vi "U3 Stream Simple Example.vi"() -> ()   [LabVIEW 2021]
panel:
  in  "Scan List (-)":u8[](array[numeric])=[31, 31, 31, 31, 31, 31, 31, 31, 31, 31, 31, 31, 31, 31, 31, 31, 31, 31, 31, 31, 31, 31, 31, 31, 31, 31, 31, 31, 31, 31, 31, 31, 31, 31, 31, 31, 31, 31, 31, 31, 31, 31, 31, 31, 31, 31, 31, 31, 31, 31, 31, 31, 31, 31, 31, 31, 31, 31, 31, 31, 31, 31, 31, 31, 31, 31, 31, 31, 31, 31, 31, 31, 31, 31, 31, 31, 31, 31, 31, 31, 31, 31, 31, 31, 31, 31, 31, 31, 31, 31, 31, 31, 31, 31, 31, 31, 31, 31, 31, 31, 31, 31, 31, 31, 31, 31, 31, 31, 31, 31, 31, 31, 31, 31, 31, 31, 31, 31, 31, 31, 31, 31, 31, 31, 31, 31, 31, 31]
  out "Waveform Graph":dbl[][](graph)
  in  "Scan List (+)":u8[](array[numeric])=[0, 1, 2, 3]
  out "Actual Scan Rate (Hz)":dbl=1000.0 format="%.3f"
  out "# Scans Read":i32
  out "# of iterations":i32
  out "Data":dbl[][](array[numeric]) format="%.3f"
  in  "Scan Rate (Hz)":dbl=1000.0 format="%.3f"
  in  "stop":bool
  out "Error Message":string
  # "This example streams from the first found USB U3.  Streaming\nrequires U3 hardware revision 1.21+."
  # "The + scan list is the positive\nchannels.  For each element in\nthe + list, there must also be\nan element in the - list, which is\nthe negative channels.  For\nsingle-ended channels, put in\n31 for the negative channel."
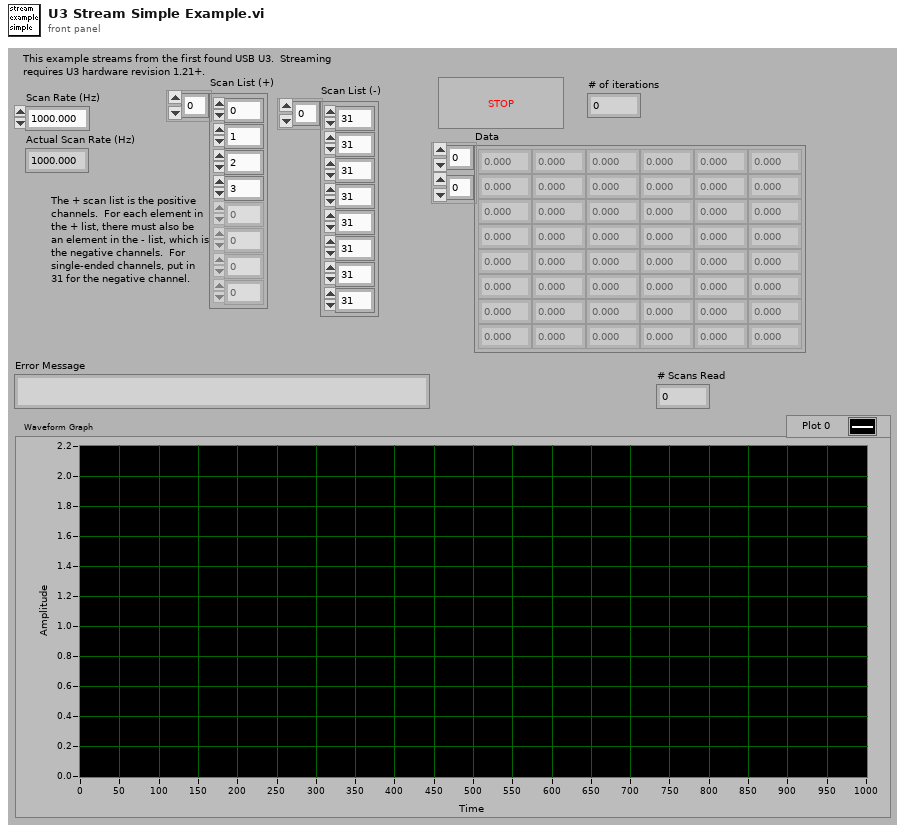
[diagram p1: front panel]
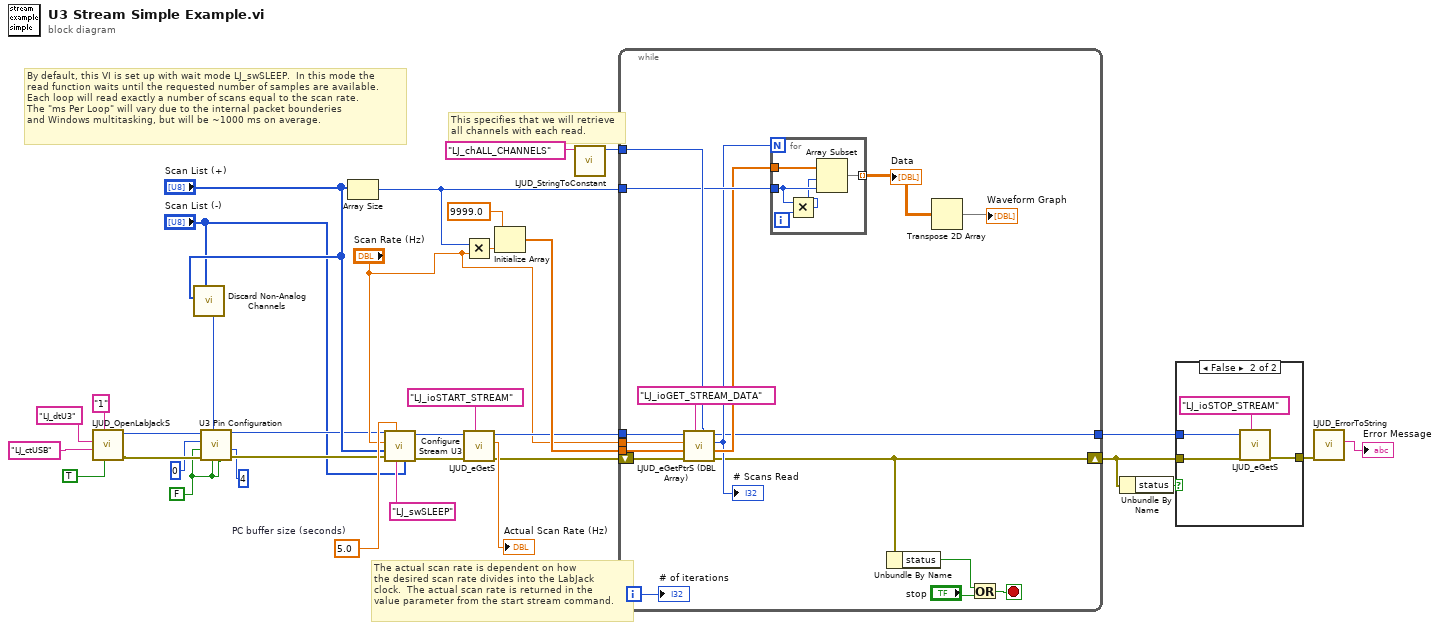
[diagram p0: block diagram]
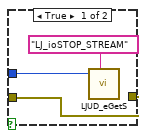
[diagram p2: hidden frame]
diagram:
  w11 = FALSE ("Enable DAC1")
  w24 = 5.0  # PC buffer size (seconds)
  # "This specifies that we will retrieve\nall channels with each read."
  # "The actual scan rate is dependent on how\nthe desired scan rate divides into the LabJack\nclock.  The actual scan rate is returned in the\nvalue parameter from the start stream command."
  # "By default, this VI is set up with wait mode LJ_swSLEEP.  In this mode the\nread function waits until the requested number of samples are available.\nEach loop will read exactly a number of scans equal to the scan rate.\nThe \"ms Per Loop\" will vary due to the internal packet bounderies\nand Windows multitasking, but will be ~1000 ms on average."
  n1 = call "LJUD_OpenLabJackS.vi"("FirstFound"=TRUE, "Address"="1", "ConnectionType"="LJ_ctUSB", "DeviceType"="LJ_dtU3") -> ("error out"=w14:errorcluster, "Handle"=w15:i32)  [unwired: 5 in, 1 out]
  n2 = call "Discard Non-Analog Channels.vi"("Channels In (-)"="Scan List (-)", "Channels In"="Scan List (+)") -> ("FIO/EIO Analog Enable"=w10:i32)  [unwired: 6 in, 3 out]
  n3 = call "U3 Pin Configuration.vi"("Timer/Counter Pin Offset"=u8 4, "Enable Counter1"=w11, "Enable Counter0"=w11, "FIO/EIO Analog Enable"=w10, "error in"=w14, "Enable DAC1"=w11, "Number of Timers Enabled"=u8 0, "Handle In"=w15) -> ("error out"=w7:errorcluster, "Handle Out"=w8:i32)  [unwired: 2 in]
  n4 = Array Size(array="Scan List (+)") -> (size(s)=w28:i32)
  n5 = call "Configure Stream U3.vi"("Scan List (-)"="Scan List (-)", "Wait Mode"="LJ_swSLEEP" ("Wait Mode (2)"), "PC buffer size (seconds)"=w24, "error in"=w7, "Scan List (+)"="Scan List (+)", "Scan Rate (Hz)"="Scan Rate (Hz)", "Handle In"=w8) -> ("error out"=w32:errorcluster, "Handle Out"=w33:i32)  [unwired: 2 in, 1 out]
  n6 = Multiply(x=w28, y="Scan Rate (Hz)") -> (x*y=w31:dbl)
  n7 = call "LJUD_eGetS.vi"("IOType"="LJ_ioSTART_STREAM", "error in"=w32, "Handle In"=w33) -> ("error out"=w17:errorcluster, "Value Read"=→"Actual Scan Rate (Hz)":dbl, "Handle Out"=w22:i32)  [unwired: 6 in]
  n8 = Initialize Array(9999.0, w31) -> (w29:dbl[])
  n9 = call "LJUD_StringToConstant.vi"("String"="LJ_chALL_CHANNELS") -> ("Constant Number"=w18:i32)  [unwired: 9 in, 1 out]
  n10 = while {
    tunnel: [w35] -> w4
    shift-left: w17 -> [w42]
    shift-right: [w36] -> w16
    tunnel: w18 -> [w43]
    tunnel: w28 -> [w39]
    tunnel: w29 -> [w46]
    tunnel: "Scan Rate (Hz)" -> [w45]
    tunnel: w22 -> [w48]
    i -> [w44]
    stop <- w49 stop-if-true
    n11 = call "LJUD_eGetPtrS (DBL Array).vi"("Channel"=w43, "IOType"="LJ_ioGET_STREAM_DATA", "error in"=w42, "DBL Array Write"=w46, "Value"=w45, "Handle In"=w48) -> ("error out"=w36:errorcluster, "DBL Array Read"=w38:dbl[], "Value"=w37:i32, "Handle Out"=w35:i32)  [unwired: 2 in]
    "# Scans Read" <- w37
    n12 = for {
      N: w37 -> [_]
      tunnel: w38 -> [w56]
      tunnel: w39 -> [w55]
      tunnel: [w52] -> w40 mode=indexing
      i -> [w54]
      n13 = Multiply(x=w55, y=w54) -> (x*y=w53:i32)
      n14 = Array Subset(array=w56, index=w53, length=w55) -> (w52:dbl[])
    }
    "Data" <- w40
    n15 = Unbundle By Name(w36) -> ("status"=w50:bool)
    n16 = Transpose 2D Array(2D array=w40) -> (transposed array=→"Waveform Graph":dbl[][])
    n17 = Or(x=w50, y="stop") -> (x .or. y?=w49:bool)
    "# of iterations" <- w44
  }
  n18 = Unbundle By Name(w16) -> ("status"=w20:bool)
  n19 = case shown="False" w20 {
    tunnel: [w58 w62] -> w26
    tunnel: w16 -> [w58 w61]
    tunnel: w4 -> [w57 w60]
    frame True {
      n20 = call "LJUD_eGetS.vi"("IOType"="LJ_ioSTOP_STREAM", "Handle In"=w57) -> ()  [unwired: 7 in, 3 out]
    }
    frame False {
      n21 = call "LJUD_eGetS.vi"("IOType"="LJ_ioSTOP_STREAM", "error in"=w61, "Handle In"=w60) -> ("error out"=w62:errorcluster)  [unwired: 6 in, 2 out]
    }
  }
  n22 = call "LJUD_ErrorToString.vi"("error in"=w26) -> ("String"=→"Error Message":string)  [unwired: 10 in]
